vi "Enqueue Main GUI Initialization.vi"(8 "error in (no error)":errorcluster, 10 "boolean reference":refnum<vi>, 11 "main gui queue":refnum<queue>) -> (0 "error out":errorcluster)   [LabVIEW 2020]
uses:
  Main GUI Loop/Handler.ctl
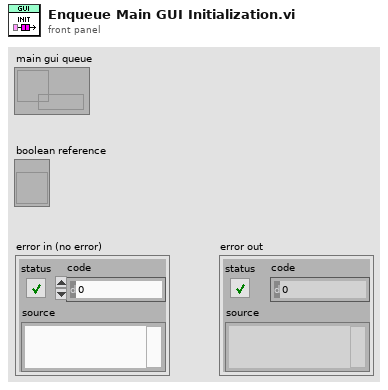
[diagram p1: front panel]
types:
  T1 = typedef "Handler.ctl" = cluster{"bool ref":refnum<vi>, "error":errorcluster, "msg":string, "status":string, "switch status":bool, "force cal":dbl[][], "force cal results":dbl[][]}
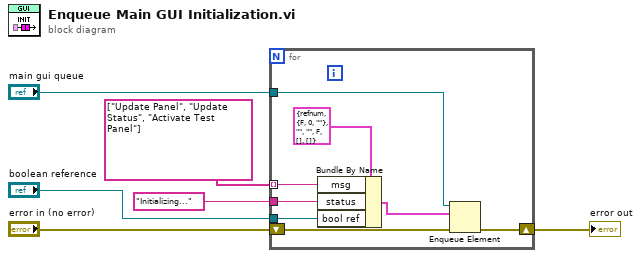
[diagram p0: block diagram]
diagram:
  n1 = for {
    tunnel: "main gui queue" -> [w14]
    tunnel: "boolean reference" -> [w12]
    tunnel: "Initializing..." ("status") -> [w11]
    shift-right: [w10] -> w5
    shift-left: "error in (no error)" -> [w13]
    tunnel: string[] ["Update Panel", "Update Status", "Activate Test Panel"] -> [w9] mode=indexing
    n2 = Bundle By Name(cluster=T1 {"bool ref"=refnum, "error"={"status"=FALSE, "code"=0, "source"=""}, "msg"="", "status"="", "switch status"=FALSE, "force cal"=[], "force cal results"=[]} ("main gui"), "msg"=w9, "status"=w11, "bool ref"=w12) -> (w7:T1)
    n3 = Enqueue Element(queue=w14, element=w7, error in (no error)=w13) -> (error out=w10:errorcluster)  [unwired: 1 in, 2 out]
  }
  "error out" <- w5
